vi "LoadWaveString.vi"(0 "Wave String":string) -> (1 "All Wave (MHz,us)":string[][](table)=[["Frequency (MHz)", "Duration (us)", "Amplitude", "Phase (Pi)", "Gap (us)"], ["200.012", "100.000", "1.000", "0.000", "0.001"]], 2 "All Wave":T1 {"Phase (Pi)" min=-1.0 max=1.0 step=0.1 format="%.2f"; "Gap (us)" format="%.2f"; "Amplitude" format="%.2f"; "Duration (us)" format="%.2f"; "Frequency (MHz)" format="%.4f"}, 3 "SegmentPositions":i32[](array[numeric]))   [LabVIEW 2014]
uses:
  Wave.ctl
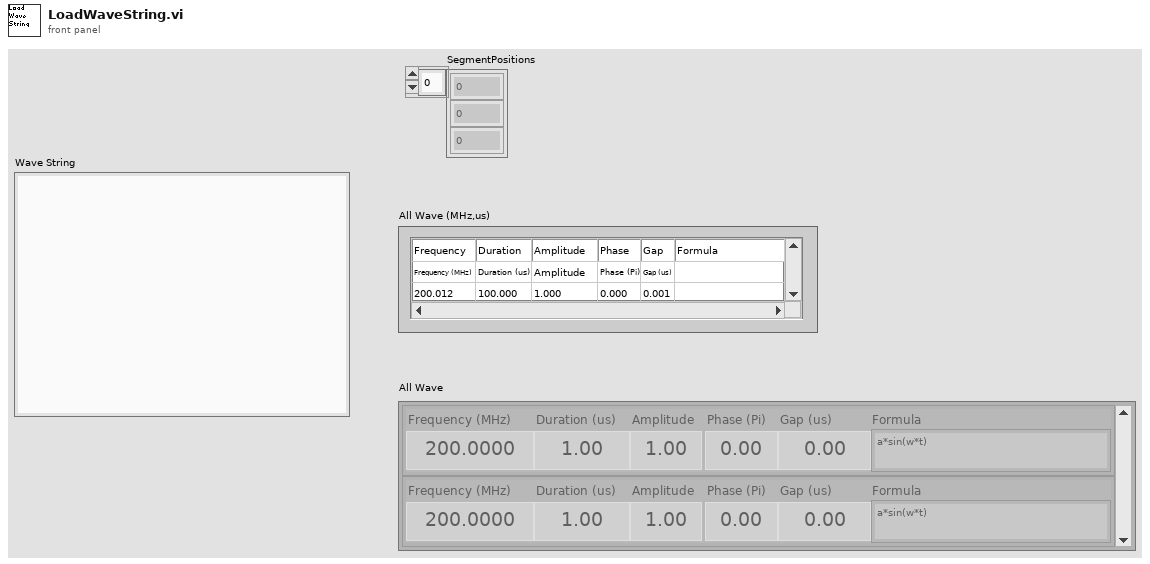
[diagram p1: front panel]
types:
  T1 = typedef "Wave.ctl" = cluster{"Frequency (MHz)":dbl, "Duration (us)":dbl, "Amplitude":dbl, "Phase (Pi)":dbl, "Gap (us)":dbl, "Formula":string}[]
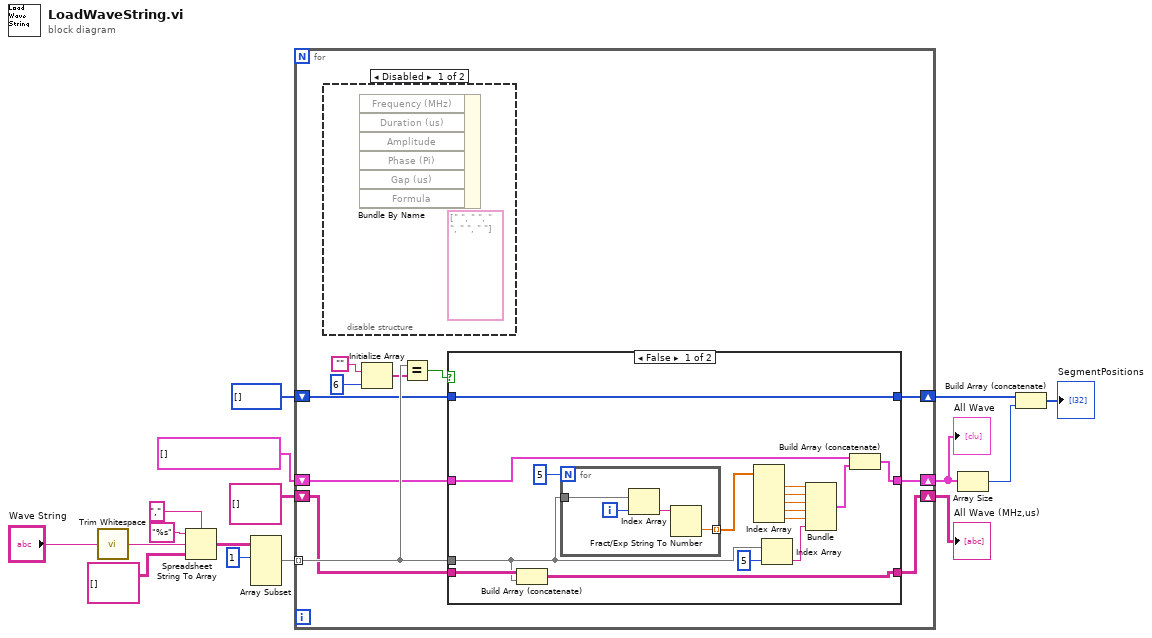
[diagram p0: block diagram]
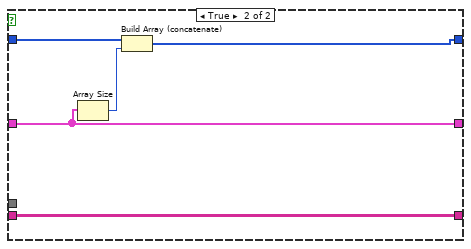
[diagram p3: hidden frame]
diagram:
  n1 = call <vilib>:"Trim Whitespace.vi"("string"="Wave String") -> ("trimmed string"=w1:string)  [unwired: 1 in]
  n2 = Spreadsheet String To Array(delimiter (Tab)="," ("delimiter (\\t)"), format string="%s", spreadsheet string=w1, array type (2D Dbl)=string[][] [] ("Wave (MHz, us, Pi)")) -> (array=w5:string[][])
  n3 = Array Subset(array=w5, index (row)=1 ("index")) -> (w3:string[][])  [unwired: 3 in]
  n4 = for {
    tunnel: w3 -> [w27] mode=indexing
    shift-right: [w22] -> w11
    shift-left: string[][] [] ("All Wave (MHz,us)") -> [w23]
    shift-right: [w20] -> w15
    shift-left: i32[] [] ("appended array") -> [w21]
    shift-right: [w17] -> w9
    shift-left: T1 [] ("All Wave") -> [w18]
    n5 = disable-structure shown="Disabled" {
      frame Disabled {
        (unwired) string[] [" ", " ", " ", " ", " "] ("y")
        n6 = Bundle By Name() -> ()  [unwired: 7 in, 1 out]
      }
      frame Enabled {
      }
    }
    n7 = Initialize Array("", 6 ("dimension size")) -> (w24:string[])
    n8 = Equal?(x=w27, y=w24) -> (x = y?=w19:bool)
    n9 = case shown="False" w19 {
      tunnel: w27 -> [w36 _]
      tunnel: [w43 w52] -> w22
      tunnel: w23 -> [w42 w52]
      tunnel: w21 -> [w41 w51]
      tunnel: [w41 w49] -> w20
      tunnel: w18 -> [w39 w48]
      tunnel: [w38 w48] -> w17
      frame False {
        n10 = Build Array (concatenate)(w42, w36) -> (w43:string[][])
        n11 = for {
          N: 5 -> [_]
          tunnel: [w47] -> w37 mode=indexing
          tunnel: w36 -> [w46]
          i -> [w45]
          n12 = Index Array(array=w46, index=w45) -> (element=w44:string)
          n13 = Fract/Exp String To Number(string=w44) -> (number=w47:dbl)  [unwired: 3 in, 1 out]
        }
        n14 = Index Array(array=w37) -> (element #1=w34:dbl, element #2=w33:dbl, element #3=w32:dbl, element #4=w31:dbl, element #5=w30:dbl)  [unwired: 5 in]
        n15 = Index Array(array=w36, index=5) -> (element=w29:string)
        n16 = Bundle(w34, w33, w32, w31, w30, w29) -> (w28:cluster{dbl, dbl, dbl, dbl, dbl, string})  [unwired: 1 in]
        n17 = Build Array (concatenate)(w39, w28) -> (w38:T1)
      }
      frame True {
        n18 = Array Size(array=w48) -> (size(s)=w50:i32)
        n19 = Build Array (concatenate)(w51, w50) -> (w49:i32[])
      }
    }
  }
  "All Wave (MHz,us)" <- w11
  "All Wave" <- w9
  n20 = Array Size(array=w9) -> (size(s)=w14:i32)
  n21 = Build Array (concatenate)(w15, w14) -> (→"SegmentPositions":i32[])
